vi "Main.vi"() -> ()   [LabVIEW 2011]
uses:
  States.ctl
panel:
  out "Execution time of Main VI (seconds)":dbl
  in  "stop":bool
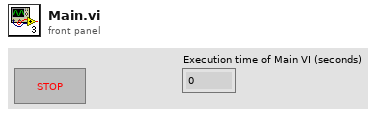
[diagram p1: front panel]
types:
  T1 = cluster{"Async VI reference":refnum<vi>, "Measurements":dbl[]}
  T2 = typedef "States.ctl" = enum16{"Initialize", "Prepare for Write", "Write", "Read", "Shutdown"}
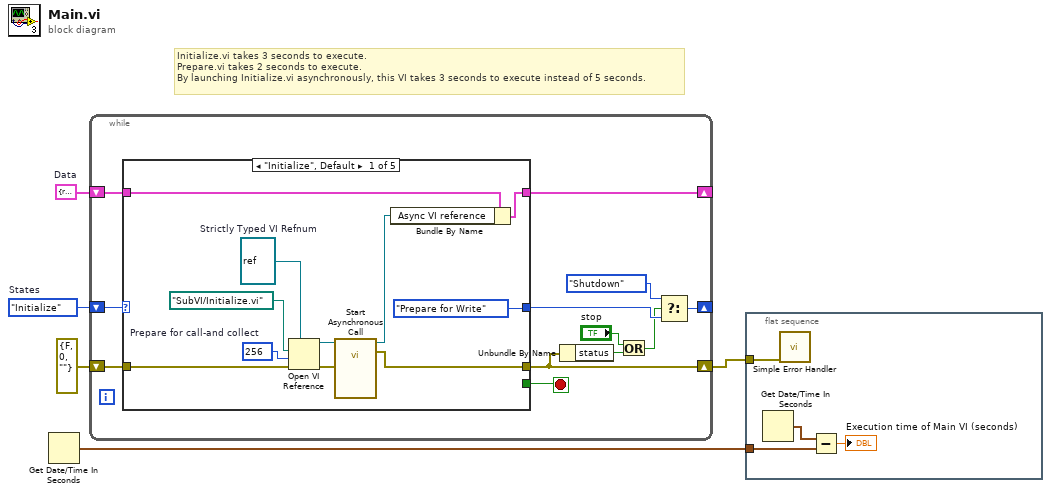
[diagram p0: block diagram]
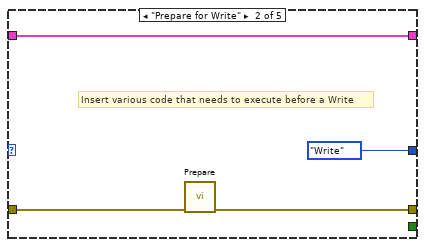
[diagram p2: hidden frame]
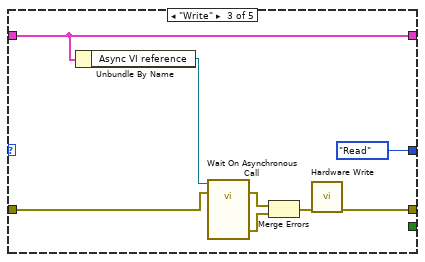
[diagram p3: hidden frame]
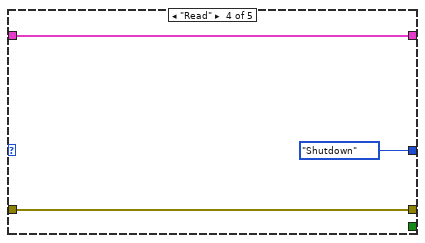
[diagram p4: hidden frame]
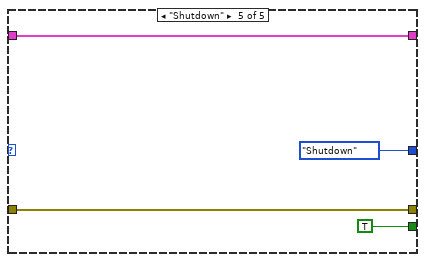
[diagram p5: hidden frame]
diagram:
  w4 = T1 {"Async VI reference"=refnum, "Measurements"=[]}  # Data
  w5 = States."Initialize"  # States
  # "Initialize.vi takes 3 seconds to execute.\nPrepare.vi takes 2 seconds to execute.\nBy launching Initialize.vi asynchronously, this VI takes 3 seconds to execute instead of 5 seconds."
  n1 = Get Date/Time In Seconds() -> (seconds since 1Jan1904=w2:timestamp)
  n2 = while {
    shift-right: [w7] -> _
    shift-left: w5 -> [w17]
    shift-right: [w15] -> _
    shift-left: w4 -> [w16]
    shift-right: [w13] -> w1
    shift-left: errorcluster {"status"=FALSE, "code"=0, "source"=""} ("error out") -> [w14]
    stop <- w6 stop-if-true
    n3 = case shown="\"Initialize\", Default" w17 {
      tunnel: w16 -> [w23 w32 w39 w43 w44]
      tunnel: [w22 w32 w39 w43 w44] -> w15
      tunnel: w14 -> [w20 w30 w37 w41 w47]
      tunnel: [w19 w29 w33 w41 w47] -> w13
      tunnel: [States."Prepare for Write" ("States") States."Write" ("States") States."Read" ("States") States."Shutdown" ("States") States."Shutdown" ("States")] -> w10
      tunnel: [_ _ _ _ TRUE] -> w6
      frame "Initialize", Default {
        w24 = 256  # Prepare for call-and collect
        w27 = refnum<vi> refnum  # Strictly Typed VI Refnum
        n4 = Open VI Reference(type specifier VI Refnum (for type only)=w27, vi path=path "SubVI/Initialize.vi", options=w24, error in (no error)=w20) -> (vi reference=w26:refnum<vi>, error out=w25:errorcluster)  [unwired: 2 in]
        n5 = call-by-ref "Start Asynchronous Call"(reference=w26, error in=w25) -> (reference out=w21:refnum<vi>, error out=w19:errorcluster)  [unwired: 11 in, 1 out]
        n6 = Bundle By Name(cluster=w23, "Async VI reference"=w21) -> (w22:T1)
      }
      frame "Prepare for Write" {
        # "Insert various code that needs to execute before a Write"
        n7 = call "Prepare.vi"("error in (no error)"=w30) -> ("error out"=w29:errorcluster)  [unwired: 10 in]
      }
      frame "Write" {
        n8 = Unbundle By Name(w39) -> ("Async VI reference"=w38:refnum<vi>)
        n9 = call-by-ref "Wait On Asynchronous Call"(reference=w38, error in=w37) -> (error out=w36:errorcluster, 0:"error out"=w35:errorcluster)  [unwired: 11 in, 1 out]
        n10 = Merge Errors(w36, w35) -> (w34:errorcluster)
        n11 = call "Hardware Write.vi"("error in (no error)"=w34) -> ("error out"=w33:errorcluster)  [unwired: 10 in]
      }
      frame "Read" {
      }
      frame "Shutdown" {
      }
    }
    n12 = Unbundle By Name(w13) -> ("status"=w12:bool)
    n13 = Or(x="stop", y=w12) -> (x .or. y?=w9:bool)
    n14 = Select(t=States."Shutdown", s=w9, f=w10) -> (s? t:f=w7:T2)
  }
  n15 = flat-sequence {
    tunnel: w1 -> [w48]
    tunnel: w2 -> [w50]
    frame #0 {
      n16 = Get Date/Time In Seconds() -> (seconds since 1Jan1904=w51:timestamp)
      n17 = call <vilib>:"Simple Error Handler.vi"("error in (no error)"=w48) -> ()  [unwired: 4 in, 5 out]
      n18 = Subtract(x=w51, y=w50) -> (x-y=→"Execution time of Main VI (seconds)":dbl)
    }
  }
